vi "Get Data.vi"(8 "error in (no error)":errorcluster, 11 "Stability Data in":refnum<class "Stability Data.lvclass">) -> (0 "error out":errorcluster, 2 "Data":cluster{"Error":sgl, "# of Obs":u16}, 3 "Stability Data out":refnum<class "Stability Data.lvclass">)   [LabVIEW 2015, in "Stability Data.lvclass"]
uses:
  Stability Data.lvclass
  Stability Data.lvclass/Stability Data.ctl
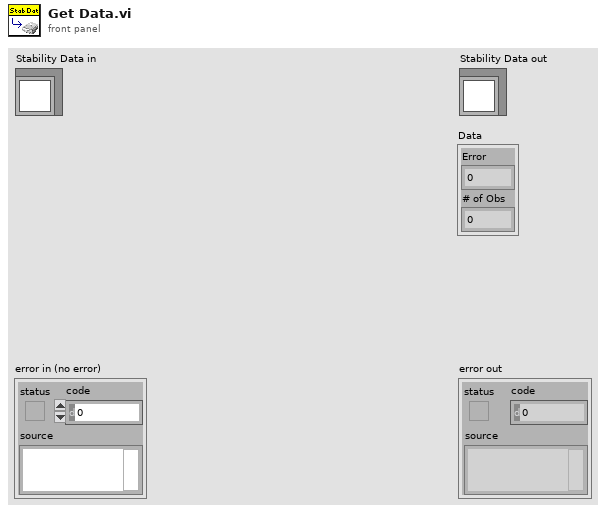
[diagram p1: front panel]
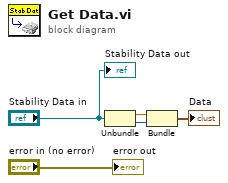
[diagram p0: block diagram]
diagram:
  n1 = Unbundle("Stability Data in") -> (w2:sgl, w1:u16)
  n2 = Bundle("Error"=w2, "# of Obs"=w1) -> (→"Data":cluster{"Error":sgl, "# of Obs":u16})  [unwired: 1 in]
  "error out" <- "error in (no error)"
  "Stability Data out" <- "Stability Data in"
